vi "Set function range value frequnecy.vi"(4 "Range number (0)":u16 max=9, 6 "Function (F0 - V DC)":T1(ring), 7 "Ignore instr. error (false)":bool, 8 "error in":errorcluster, 9 "Frequency [Hz]":dbl=10.0 min=10.0 max=1000000.0, 10 "Value":dbl, 11 "VISA resource name":refnum<visa-resource-name>) -> (0 "error out":errorcluster, 2 "Setup failed":bool, 3 "VISA resource name out":refnum<visa-resource-name>)   [LabVIEW 2013, in "Datron D4xxx.lvlib"]
doc: "This VI sets calls \"set function and range\" and \"set value and frequency\" VIs. Options are same as for theese VIs."
uses:
  Datron D4xxx.lvlib
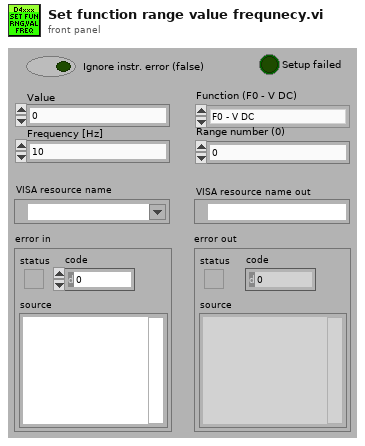
[diagram p1: front panel]
types:
  T1 = enum16{"F0 - V DC", "F1 - V AC", "F2 - A DC", "F3 - A AC", "F4 - R", "F5 - V WB"}
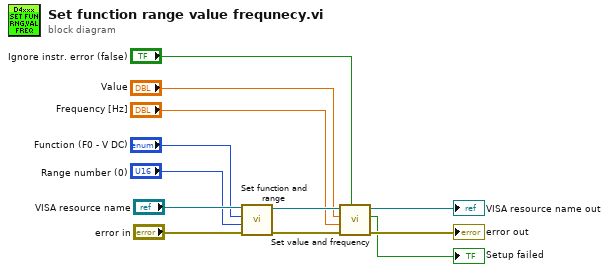
[diagram p0: block diagram]
diagram:
  n1 = call "Set function and range.vi"("error in"="error in", "Range number (0)"="Range number (0)", "Function (F0 - V DC)"="Function (F0 - V DC)", "VISA resource name"="VISA resource name") -> ("error out"=w10:errorcluster, "VISA resource name out"=w9:refnum<visa-resource-name>)  [unwired: 6 in]
  n2 = call "Set value and frequency.vi"("Ignore instr. error (false)"="Ignore instr. error (false)", "error in"=w10, "Frequency [Hz]"="Frequency [Hz]", "Value"="Value", "VISA resource name"=w9) -> ("error out"=→"error out":errorcluster, "Setup failed"=→"Setup failed":bool, "VISA resource name out"=→"VISA resource name out":refnum<visa-resource-name>)  [unwired: 4 in]
